vi "20211224_HW2.vi"() -> ()   [LabVIEW 2019]
uses:
  Info.ctl
  <vilib>/Utility/miscctls.llb/LVPositionTypeDef.ctl
  Status.ctl
  Motion_Info.ctl
panel:
  out "Deg":dbl
  out "Ball":bool
  out "2D Picture":picture
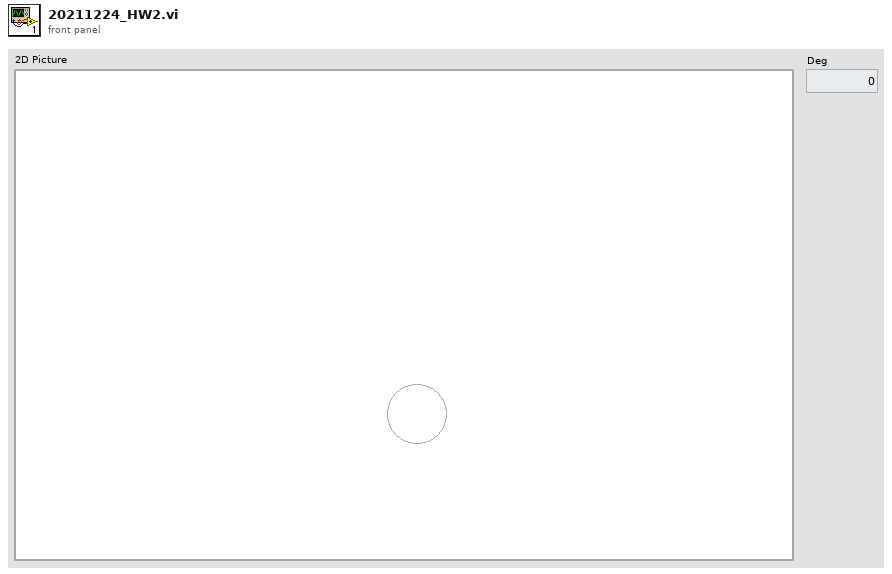
[diagram p1: front panel]
types:
  T1 = typedef "Motion_Info.ctl" = cluster{"Start Theta":dbl, "Period":dbl, "Start Time":u32}
  T2 = typedef "Status.ctl" = enum16{"Idle", "Motion"}
  T3 = cluster{"Width":u16, "Style":enum32{"Solid", "Dash", "Dot", "DashDot", "DashDotDot"}}
  T4 = typedef "LVPositionTypeDef.ctl" = cluster{"Left":i32, "Top":i32}
  T5 = typedef "Info.ctl" = cluster{"Start Drag":bool, "Position Offset":T4, "Theta Offset":dbl}
  T6 = typedef "LVBoundsTypeDef.ctl" = cluster{"Width":u32, "Height":u32}
  T7 = typedef "LVPoint32TypeDef.ctl" = cluster{"Horizontal":i32, "Vertical":i32}
  T8 = cluster{"Label.Bounds:Area Height":u32, "Label.Height":u32}
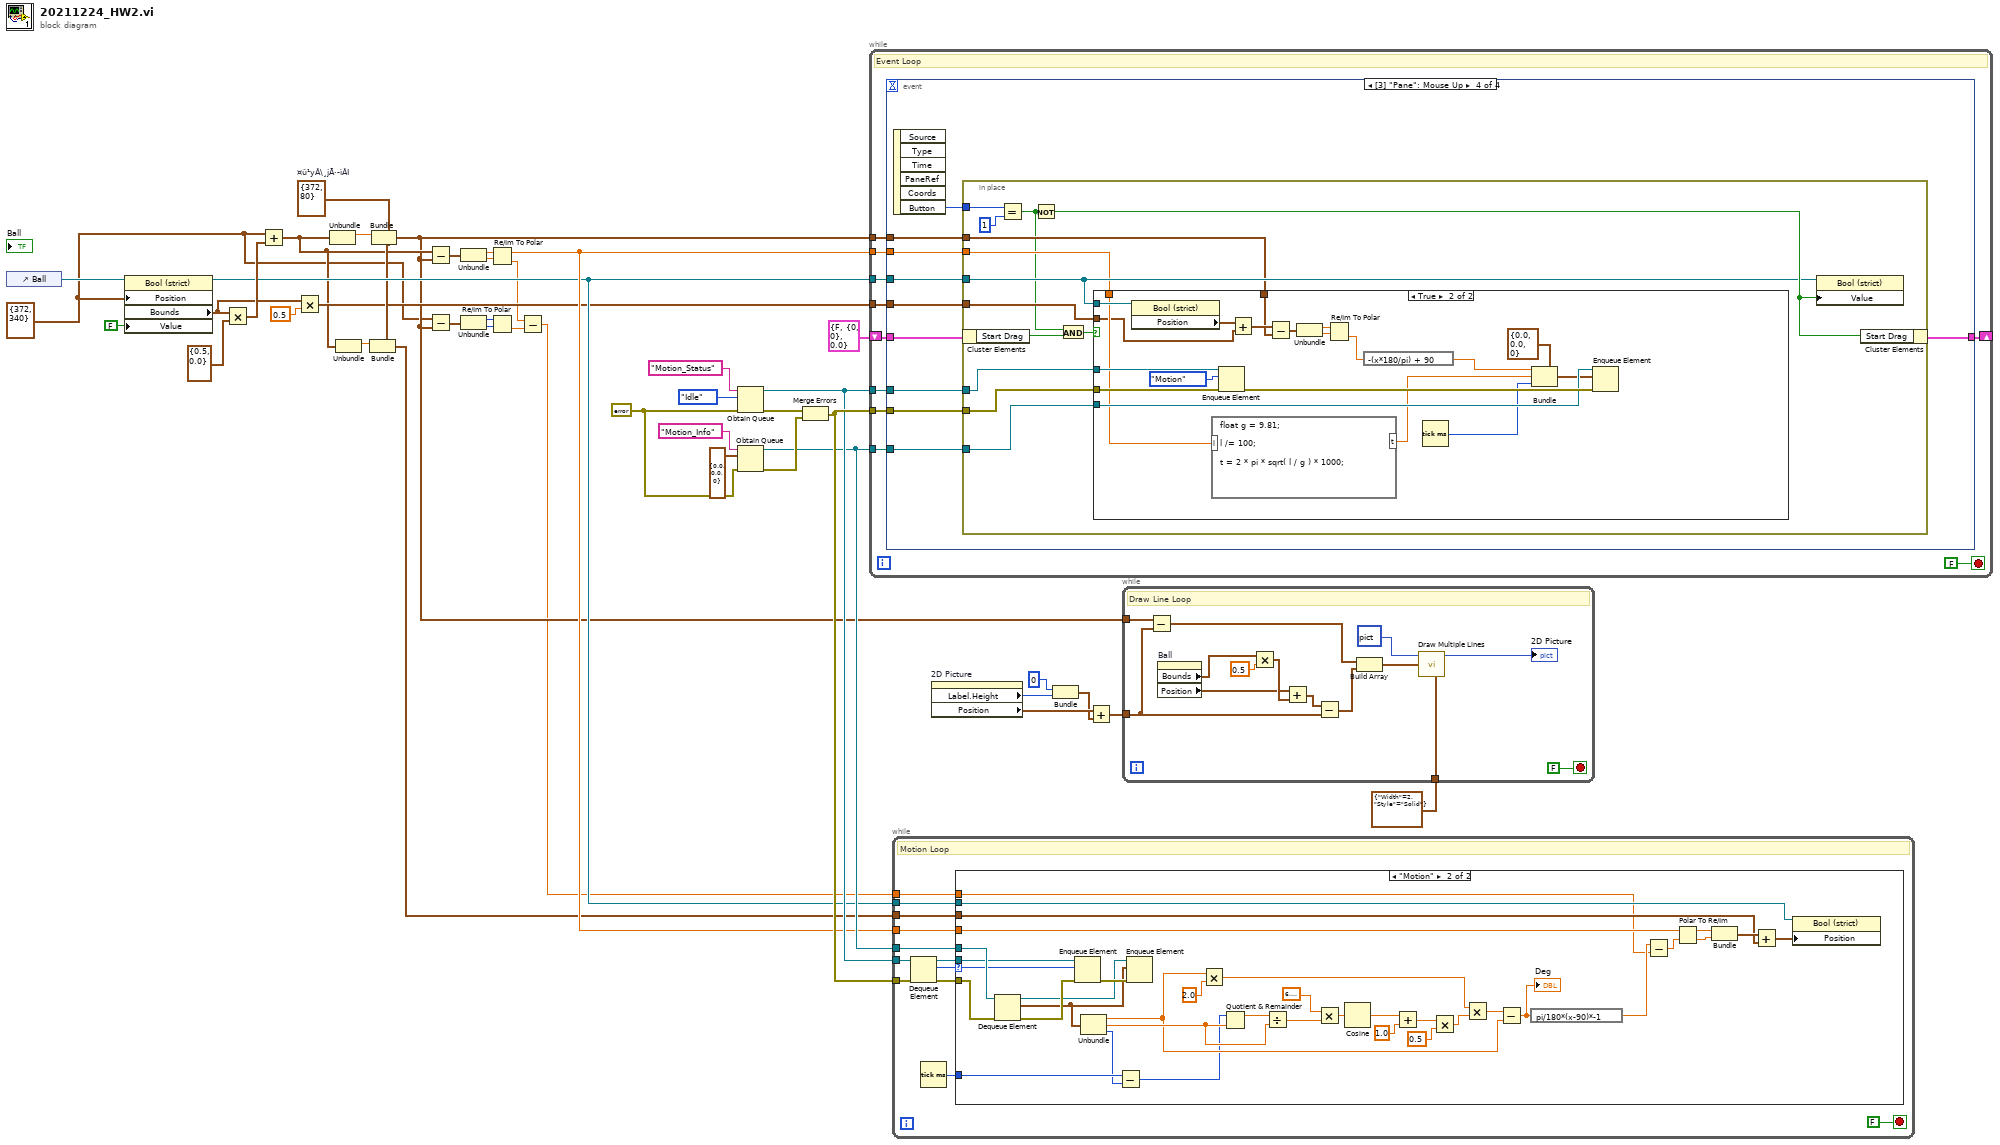
[diagram p0: block diagram]
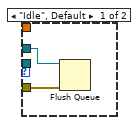
[diagram p2: hidden frame]
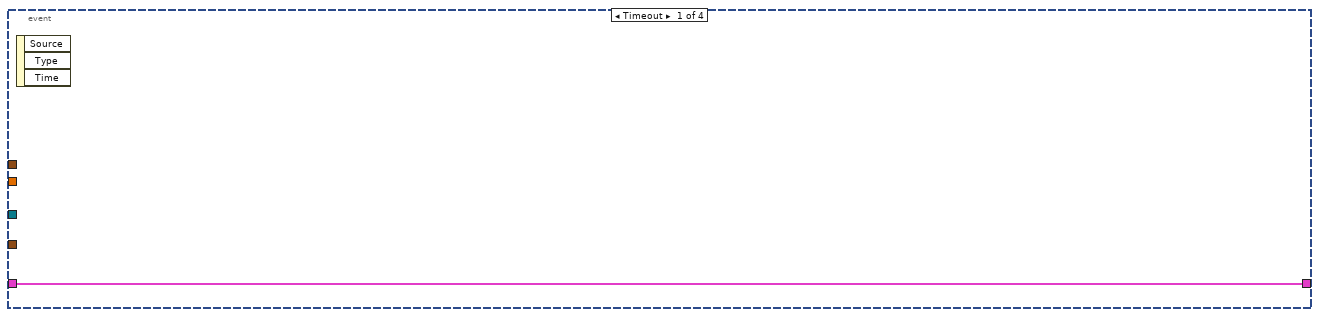
[diagram p3: hidden frame]
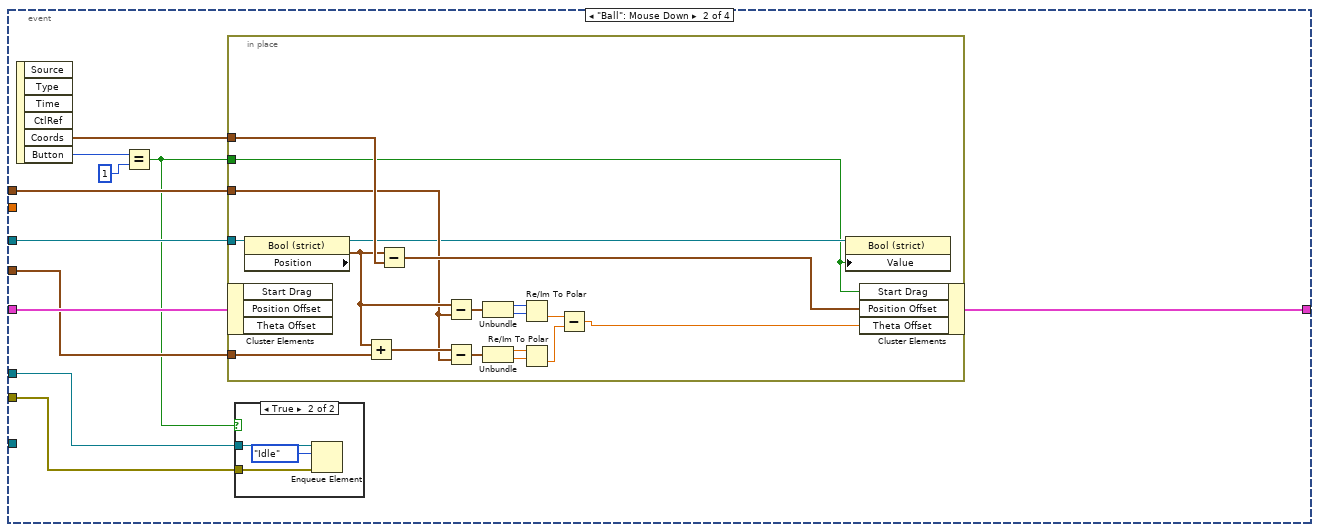
[diagram p4: hidden frame]
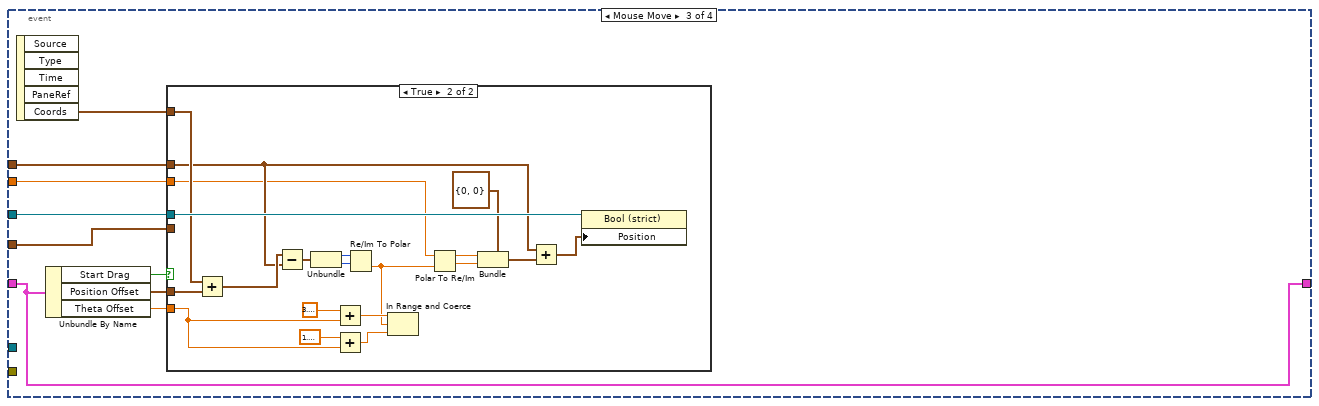
[diagram p6: hidden frame]
diagram:
  w22 = errorcluster {"status"=FALSE, "code"=0, "source"=""} ("error in (no error)")
  w13 = T4 {"Left"=372, "Top"=80}  # ¤û¹yÂ\¸jÃ·­ìÂI
  w5 = T4 {"Left"=372, "Top"=340} ("Position")
  n1 = control-ref of="Ball"() -> (w41:refnum<vi>)
  n2 = property class="Bool (strict)"(reference=w41, "Position"=w5, "Value"=FALSE) -> (reference out=w14:refnum<vi>, "Bounds"=w33:T6)  [unwired: 1 in, 1 out]
  n3 = Multiply(x=w33, y=cluster{"Width":dbl, "Height":dbl} {"Width"=0.5, "Height"=0.0}) -> (x*y=w34:cluster{"Width":dbl, "Height":dbl})
  n4 = Add(x=w5, y=w34) -> (x+y=w11:cluster{dbl, dbl})
  n5 = Multiply(x=w33, y=0.5 ("Width")) -> (x*y=w12:cluster{"Width":dbl, "Height":dbl})
  n6 = Unbundle(w11) -> (w40:dbl)  [unwired: 1 out]
  n7 = Unbundle(w11) -> (w10:dbl)  [unwired: 1 out]
  n8 = Bundle(cluster=w13, "Left"=w10) -> (w9:T4)  [unwired: 1 in]
  n9 = Bundle(cluster=w13, "Left"=w40) -> (w6:T4)  [unwired: 1 in]
  n10 = Subtract(x=w11, y=w6) -> (x-y=w36:cluster{dbl, dbl})
  n11 = Subtract(x=w5, y=w6) -> (x-y=w8:T4)
  n12 = Unbundle(w36) -> (w37:dbl, w38:dbl)
  n13 = Unbundle(w8) -> ("Left"=w1:i32, "Top"=w7:i32)
  n14 = Re/Im To Polar(2:w38, 3:w37) -> (0:w4:dbl, 1:w15:dbl)
  n15 = Re/Im To Polar(2:w7, 3:w1) -> (0:w3:dbl)  [unwired: 1 out]
  n16 = Subtract(x=w4, y=w3) -> (x-y=w2:dbl)
  n17 = Obtain Queue(name (unnamed)="Motion_Status", element data type=Status."Idle", error in (no error)=w22) -> (queue out=w17:refnum<queue>, error out=w20:errorcluster)  [unwired: 2 in, 1 out]
  n18 = Obtain Queue(name (unnamed)="Motion_Info", element data type=T1 {"Start Theta"=0.0, "Period"=0.0, "Start Time"=0}, error in (no error)=w22) -> (queue out=w16:refnum<queue>, error out=w19:errorcluster)  [unwired: 2 in, 1 out]
  n19 = Merge Errors(w20, w19) -> (w18:errorcluster)
  n20 = while {
    shift-right: [w49] -> _
    shift-left: T5 {"Start Drag"=FALSE, "Position Offset"={"Left"=0, "Top"=0}, "Theta Offset"=0.0} -> [w51]
    tunnel: w14 -> [w50]
    tunnel: w6 -> [w48]
    tunnel: w15 -> [w47]
    tunnel: w12 -> [w46]
    tunnel: w18 -> [w45]
    tunnel: w17 -> [w44]
    tunnel: w16 -> [w43]
    stop <- FALSE stop-if-true
    # "Event Loop"
    n21 = event shown="[3] \"Pane\": Mouse Up" {
      selector: _ -> [_ _ _ _]
      dyn-events: _ -> [_ _ _ _]
      timeout: _ -> [_ _ _ _]
      tunnel: w51 -> [w53 w64 w90 w123]
      tunnel: w50 -> [_ w62 w94 w121]
      tunnel: [w53 w63 w90 w122] -> w49
      tunnel: w48 -> [_ w60 w89 w117]
      tunnel: w47 -> [_ _ w88 w115]
      tunnel: w46 -> [_ w59 w87 w116]
      tunnel: w45 -> [_ w55 _ w120]
      tunnel: w44 -> [_ w54 _ w119]
      tunnel: w43 -> [_ _ _ w118]
      event Timeout {
        n22 = event-data() -> ()  [unwired: 1 in, 3 out]
      }
      event "Ball": Mouse Down {
        n23 = event-data() -> ("Coords"=w61:T7, "Button"=w57:u16)  [unwired: 1 in, 4 out]
        n24 = Equal?(x=w57, y=u16 1) -> (x = y?=w56:bool)
        n25 = in-place {
          in-place-border: w62 -> [w85]
          in-place-border: w61 -> [w84]
          in-place-border: w60 -> [w76]
          in-place-border: w59 -> [w79]
          in-place-border: w56 -> [w68]
          n26 = in-place-cluster #1(w64) -> ()  [unwired: 3 out]
          n27 = property class="Bool (strict)"(reference=w85) -> (reference out=w69:refnum<vi>, "Position"=w80:T4)  [unwired: 1 in, 1 out]
          n28 = Add(x=w80, y=w79) -> (x+y=w77:cluster{dbl, dbl})
          n29 = Subtract(x=w80, y=w84) -> (x-y=w81:T4)
          n30 = Subtract(x=w80, y=w76) -> (x-y=w78:T4)
          n31 = Subtract(x=w77, y=w76) -> (x-y=w75:cluster{dbl, dbl})
          n32 = Unbundle(w78) -> ("Left"=w83:i32, "Top"=w82:i32)
          n33 = Unbundle(w75) -> (w74:dbl, w73:dbl)
          n34 = Re/Im To Polar(2:w82, 3:w83) -> (0:w72:dbl)  [unwired: 1 out]
          n35 = Re/Im To Polar(2:w73, 3:w74) -> (0:w71:dbl)  [unwired: 1 out]
          n36 = Subtract(x=w72, y=w71) -> (x-y=w70:dbl)
          n37 = property class="Bool (strict)"(reference=w69, "Value"=w68) -> ()  [unwired: 1 in, 2 out]
          n38 = in-place-cluster #1("Start Drag"=w68, "Position Offset"=w81, "Theta Offset"=w70) -> (w63:T5)
        }
        n39 = case shown="True" w56 {
          tunnel: w55 -> [_ w66]
          tunnel: w54 -> [_ w65]
          frame False {
          }
          frame True {
            n40 = Enqueue Element(queue=w65, element=Status."Idle", error in (no error)=w66) -> ()  [unwired: 1 in, 3 out]
          }
        }
      }
      event Mouse Move {
        n41 = event-data() -> ("Coords"=w93:T7)  [unwired: 1 in, 4 out]
        n42 = Unbundle By Name(w90) -> ("Start Drag"=w92:bool, "Position Offset"=w91:T4, "Theta Offset"=w86:dbl)
        n43 = case shown="True" w92 {
          tunnel: w94 -> [_ w114]
          tunnel: w93 -> [_ w110]
          tunnel: w91 -> [_ w108]
          tunnel: w89 -> [_ w103]
          tunnel: w88 -> [_ w102]
          tunnel: w87 -> [_ _]
          tunnel: w86 -> [_ w98]
          frame False {
          }
          frame True {
            n44 = Add(x=w110, y=w108) -> (x+y=w109:T7)
            n45 = Subtract(x=w109, y=w103) -> (x-y=w113:T7)
            n46 = Unbundle(w113) -> ("Horizontal"=w112:i32, "Vertical"=w111:i32)
            n47 = Add(x=3.141592653589793, y=w98) -> (x+y=w97:dbl)
            n48 = Add(x=1.5707963267948966, y=w98) -> (x+y=w96:dbl)
            n49 = Re/Im To Polar(2:w111, 3:w112) -> (0:w95:dbl)  [unwired: 1 out]
            n50 = In Range and Coerce(upper limit=w97, x=w95, lower limit=w96) -> ()  [unwired: 2 out]
            n51 = Polar To Re/Im(2:w95, 3:w102) -> (0:w106:dbl, 1:w107:dbl)
            n52 = Bundle(cluster=T4 {"Left"=0, "Top"=0} ("Position"), "Left"=w107, "Top"=w106) -> (w105:T4)
            n53 = Add(x=w103, y=w105) -> (x+y=w101:T4)
            n54 = property class="Bool (strict)"(reference=w114, "Position"=w101) -> ()  [unwired: 1 in, 2 out]
          }
        }
      }
      event Mouse Up {
        n55 = event-data() -> ("Button"=w124:u16)  [unwired: 1 in, 5 out]
        n56 = in-place {
          in-place-border: w124 -> [w137]
          in-place-border: w121 -> [w129]
          in-place-border: w120 -> [w133]
          in-place-border: w119 -> [w132]
          in-place-border: w118 -> [w130]
          in-place-border: w117 -> [w127]
          in-place-border: w116 -> [w128]
          in-place-border: w115 -> [w126]
          n57 = in-place-cluster #2(w123) -> ("Start Drag"=w135:bool)
          n58 = Equal?(x=w137, y=u16 1) -> (x = y?=w125:bool)
          n59 = Not(x=w125) -> (.not. x?=w134:bool)
          n60 = And(x=w125, y=w135) -> (x .and. y?=w131:bool)
          n61 = case shown="True" w131 {
            tunnel: w133 -> [_ w157]
            tunnel: w132 -> [_ w156]
            tunnel: w130 -> [_ w153]
            tunnel: w129 -> [_ w152]
            tunnel: w128 -> [_ w138]
            tunnel: w127 -> [_ w149]
            tunnel: w126 -> [_ w143]
            frame False {
            }
            frame True {
              n62 = property class="Bool (strict)"(reference=w152) -> ("Position"=w151:T4)  [unwired: 1 in, 2 out]
              n63 = formula code="float g = 9.81;\n\nl /= 100;\n\nt = 2 * pi * sqrt( l / g ) * 1000;"("l"=w143) -> ("t"=w142:dbl)
              n64 = Enqueue Element(queue=w156, element=Status."Motion", error in (no error)=w157) -> (error out=w154:errorcluster)  [unwired: 1 in, 2 out]
              n65 = Add(x=w151, y=w138) -> (x+y=w150:cluster{dbl, dbl})
              n66 = Subtract(x=w150, y=w149) -> (x-y=w148:cluster{dbl, dbl})
              n67 = Unbundle(w148) -> (w147:dbl, w146:dbl)
              n68 = Re/Im To Polar(2:w146, 3:w147) -> (0:w140:dbl)  [unwired: 1 out]
              n69 = expression code="-(x*180/pi) + 90"(w140) -> (w139:dbl)
              n70 = Tick Count (ms)() -> (millisecond timer value=w141:u32)
              n71 = Bundle(cluster=T1 {"Start Theta"=0.0, "Period"=0.0, "Start Time"=0}, "Start Theta"=w139, "Period"=w142, "Start Time"=w141) -> (w144:T1)
              n72 = Enqueue Element(queue=w153, element=w144, error in (no error)=w154) -> ()  [unwired: 1 in, 3 out]
            }
          }
          n73 = property class="Bool (strict)"(reference=w129, "Value"=w134) -> ()  [unwired: 1 in, 2 out]
          n74 = in-place-cluster #2("Start Drag"=w134) -> (w122:T5)
        }
      }
    }
  }
  n75 = while {
    tunnel: w18 -> [w169]
    tunnel: w17 -> [w168]
    tunnel: w16 -> [w164]
    tunnel: w15 -> [w161]
    tunnel: w9 -> [w160]
    tunnel: w14 -> [w159]
    tunnel: w2 -> [w158]
    stop <- FALSE stop-if-true
    # "Motion Loop"
    n76 = Dequeue Element(queue=w168, error in (no error)=w169) -> (queue out=w163:refnum<queue>, element=w166:T2, error out=w165:errorcluster)  [unwired: 1 in, 1 out]
    n77 = Tick Count (ms)() -> (millisecond timer value=w162:u32)
    n78 = case shown="\"Motion\"" w166 {
      selector: w166 -> [_ w201]
      tunnel: w165 -> [w171 w207]
      tunnel: w164 -> [w170 w206]
      tunnel: w163 -> [_ w204]
      tunnel: w162 -> [_ w200]
      tunnel: w161 -> [_ w190]
      tunnel: w160 -> [_ w186]
      tunnel: w159 -> [_ w184]
      tunnel: w158 -> [_ w172]
      frame "Idle", Default {
        n79 = Flush Queue(queue=w170, error in (no error)=w171) -> ()  [unwired: 3 out]
      }
      frame "Motion" {
        n80 = Dequeue Element(queue=w206, error in (no error)=w207) -> (queue out=w202:refnum<queue>, element=w199:T1, error out=w205:errorcluster)  [unwired: 1 in, 1 out]
        n81 = Enqueue Element(queue=w204, element=w201, error in (no error)=w205) -> (error out=w203:errorcluster)  [unwired: 1 in, 2 out]
        n82 = Unbundle(w199) -> ("Start Theta"=w191:dbl, "Period"=w197:dbl, "Start Time"=w198:u32)
        n83 = Subtract(x=w200, y=w198) -> (x-y=w181:u32)
        n84 = Enqueue Element(queue=w202, element=w199, error in (no error)=w203) -> ()  [unwired: 1 in, 3 out]
        n85 = Multiply(x=w191, y=2.0) -> (x*y=w180:dbl)
        n86 = Quotient & Remainder(x=w181, y=w197) -> (x-y*floor(x/y)=w182:dbl)  [unwired: 1 out]
        n87 = Divide(x=w182, y=w197) -> (x/y=w195:dbl)
        n88 = Multiply(x=6.283185307179586, y=w195) -> (x*y=w194:dbl)
        n89 = Cosine(x=w194) -> (cos(x)=w179:dbl)
        n90 = Add(x=w179, y=1.0) -> (x+y=w177:dbl)
        n91 = Multiply(x=w177, y=0.5) -> (x*y=w175:dbl)
        n92 = Multiply(x=w180, y=w175) -> (x*y=w192:dbl)
        n93 = Subtract(x=w192, y=w191) -> (x-y=w183:dbl)
        "Deg" <- w183
        n94 = expression code="pi/180*(x-90)*-1"(w183) -> (w174:dbl)
        n95 = Subtract(x=w174, y=w172) -> (x-y=w173:dbl)
        n96 = Polar To Re/Im(2:w173, 3:w190) -> (0:w188:dbl, 1:w189:dbl)
        n97 = Bundle(w189, w188) -> (w187:cluster{dbl, dbl})  [unwired: 1 in]
        n98 = Add(x=w187, y=w186) -> (x+y=w185:cluster{dbl, dbl})
        n99 = property class="Bool (strict)"(reference=w184, "Position"=w185) -> ()  [unwired: 1 in, 2 out]
      }
    }
  }
  n100 = property on="2D Picture" class="Pict"() -> ("Label.Height"=w31:u32, "Position"=w29:T4)  [unwired: 2 in, 2 out]
  n101 = Bundle("Label.Bounds:Area Height"=u32 0, "Label.Height"=w31) -> (w28:T8)  [unwired: 1 in]
  n102 = Add(x=w29, y=w28) -> (x+y=w27:cluster{u32, u32})
  n103 = while {
    tunnel: w6 -> [w216]
    tunnel: w27 -> [w210]
    tunnel: T3 {"Width"=2, "Style"=enum."Solid"} ("pen") -> [w214]
    stop <- FALSE stop-if-true
    # "Draw Line Loop"
    n104 = Subtract(x=w216, y=w210) -> (x-y=w215:cluster{u32, u32})
    n105 = property on="Ball" class="Bool (strict)"() -> ("Bounds"=w211:T6, "Position"=w209:T4)  [unwired: 2 in, 2 out]
    n106 = Multiply(x=w211, y=0.5 ("Width")) -> (x*y=w218:cluster{"Width":dbl, "Height":dbl})
    n107 = Add(x=w209, y=w218) -> (x+y=w208:cluster{dbl, dbl})
    n108 = Subtract(x=w208, y=w210) -> (x-y=w212:cluster{dbl, dbl})
    n109 = Build Array(w215, w212) -> (w217:cluster{dbl, dbl}[])
    n110 = call <vilib>:"Draw Multiple Lines.vi"("picture"=picture data[5B], "line endpoints"=w217, "pen"=w214) -> ("new picture"=→"2D Picture":picture)  [unwired: 6 in]
  }
